vi "Synth Freq to Word.vi"(11 "Frequency (Hz)":dbl format="%#_9p") -> (1 "Actual frequency, Hz":ext format="%_20p", 2 "Freq step":ext format="%_20p", 3 "f-word out":u32)   [LabVIEW 2015]
doc: "Converts floating point frequency in Hz to 32-bit chip-programming word"
panel:
  # "Converts floating point frequency in Hz to 32-bit chip-programming word"
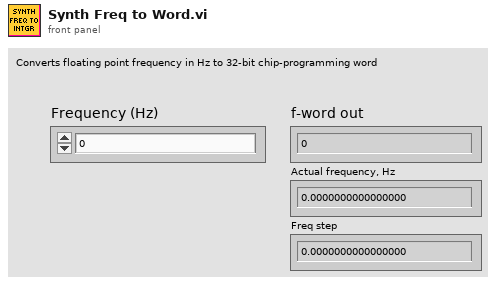
[diagram p1: front panel]
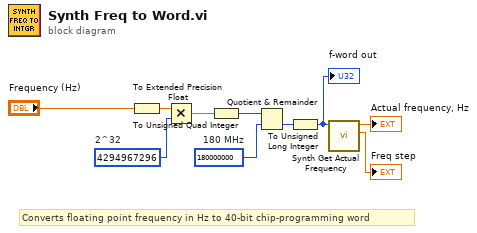
[diagram p0: block diagram]
diagram:
  w4 = u64 4294967296  # 2^32
  w6 = u64 180000000  # 180 MHz
  # "Converts floating point frequency in Hz to 40-bit chip-programming word"
  n1 = To Extended Precision Float(1:"Frequency (Hz)") -> (0:w7:ext)
  n2 = Multiply(x=w7, y=w4) -> (x*y=w9:ext)
  n3 = To Unsigned Quad Integer(1:w9) -> (0:w5:u64)
  n4 = Quotient & Remainder(x=w5, y=w6) -> (floor(x/y)=w10:u64)  [unwired: 1 out]
  n5 = To Unsigned Long Integer(number=w10) -> (unsigned 32bit integer=w3:u32)
  "f-word out" <- w3
  n6 = call "Synth Get Actual Frequency.vi"("f-word"=w3) -> ("Freq step"=→"Freq step":ext, "Actual frequency, Hz"=→"Actual frequency, Hz":ext)  [unwired: 9 in]
